vi "Multify(CDB).vi"(1 "启用（T）":bool=TRUE, 2 "In":cdb, 4 "n":cdb=1.0+0.0i) -> (6 "Out":cdb=1.0+0.0i format="%.2f")   [LabVIEW 2011]
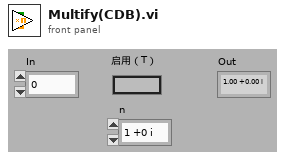
[diagram p1: front panel]
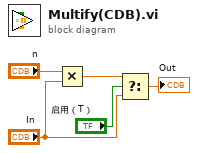
[diagram p0: block diagram]
diagram:
  n1 = Multiply(x="n", y="In") -> (x*y=w1:cdb)
  n2 = Select(t=w1, s="启用（T）", f="In") -> (s? t:f=→"Out":cdb)
